vi "Проверка работоспособности.vi"() -> ()   [LabVIEW 2013]
uses:
  IS-95/transmitter/4800/coding(4800).vi
  IS-95/transmitter/common/interleaver.vi
  IS-95/transmitter/9600/coding(9600).vi
  <vilib>/Analysis/baseanly.llb/A x B.vi
  <vilib>/Analysis/baseanly.llb/Real A x B.vi
  IS-95/transmitter/4800/syndrom(4800).vi
  IS-95/transmitter/9600/syndrom(9600).vi
  <vilib>/Analysis/Matrix/Numeric/Conversions/Array To Matrix.vi
  <vilib>/Analysis/Matrix/Numeric/Conversions/Array To Matrix - RA.vi
  <vilib>/ptbypt/Other Functions.llb/Complex Queue PtByPt.vi
panel:
  in  "Номер\nканала":i32
  in  "stop":bool
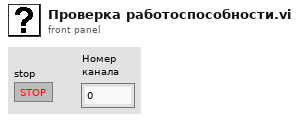
[diagram p1: front panel]
types:
  T1 = cluster{"Amplitude":dbl, "Number":i32, "Frame":bool[], "Type":i32}
  T2 = cluster{"Amplitude":dbl, "Number":i32, "Frame":bool[], "Type":i32}[]
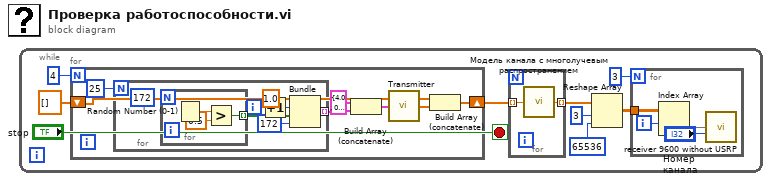
[diagram p0: block diagram]
diagram:
  n1 = while {
    stop <- "stop" stop-if-true
    n2 = for {
      N: 4 -> [_]
      shift-right: [w17] -> w6
      shift-left: cdb[] [] -> [w16]
      n3 = for {
        N: 25 -> [_]
        tunnel: [w25] -> w21 mode=indexing
        i -> [w26]
        n4 = for {
          N: 172 -> [_]
          tunnel: [w30] -> w24 mode=indexing
          n5 = Random Number (0-1)() -> (number: 0 to 1=w32:dbl)
          n6 = Greater?(x=w32, y=0.5) -> (0:w30:bool)
        }
        n7 = Increment(x=w26) -> (x+1=w27:i32)
        n8 = Bundle(1.0, w27, w24, 172) -> (w25:cluster{dbl, i32, bool[], i32})  [unwired: 1 in]
      }
      n9 = Build Array (concatenate)(T1 {"Amplitude"=4.0, "Number"=0, "Frame"=[FALSE, FALSE, FALSE, FALSE, FALSE, FALSE, FALSE, FALSE, FALSE, FALSE, FALSE, FALSE, FALSE, FALSE, FALSE, FALSE, FALSE, FALSE, FALSE, FALSE, FALSE, FALSE, FALSE, FALSE, FALSE, FALSE, FALSE, FALSE, FALSE, FALSE, FALSE, FALSE, FALSE, FALSE, FALSE, FALSE, FALSE, FALSE, FALSE, FALSE, FALSE, FALSE, FALSE, FALSE, FALSE, FALSE, FALSE, FALSE, FALSE, FALSE, FALSE, FALSE, FALSE, FALSE, FALSE, FALSE, FALSE, FALSE, FALSE, FALSE, FALSE, FALSE, FALSE, FALSE, FALSE, FALSE, FALSE, FALSE, FALSE, FALSE, FALSE, FALSE, FALSE, FALSE, FALSE, FALSE, FALSE, FALSE, FALSE, FALSE, FALSE, FALSE, FALSE, FALSE, FALSE, FALSE, FALSE, FALSE, FALSE, FALSE, FALSE, FALSE, FALSE, FALSE, FALSE, FALSE, FALSE, FALSE, FALSE, FALSE, FALSE, FALSE, FALSE, FALSE, FALSE, FALSE, FALSE, FALSE, FALSE, FALSE, FALSE, FALSE, FALSE, FALSE, FALSE, FALSE, FALSE, FALSE, FALSE, FALSE, FALSE, FALSE, FALSE, FALSE, FALSE, FALSE, FALSE, FALSE, FALSE, FALSE, FALSE, FALSE, FALSE, FALSE, FALSE, FALSE, FALSE, FALSE, FALSE, FALSE, FALSE, FALSE, FALSE, FALSE, FALSE, FALSE, FALSE, FALSE, FALSE, FALSE, FALSE, FALSE, FALSE, FALSE, FALSE, FALSE, FALSE, FALSE, FALSE, FALSE, FALSE, FALSE, FALSE, FALSE, FALSE, FALSE, FALSE, FALSE, FALSE, FALSE, FALSE, FALSE], "Type"=172} ("Cluster"), w21) -> (w19:T2)
      n10 = call "Transmitter.vi"("CHANNELS"=w19) -> ("x + iy"=w18:cdb[])  [unwired: 14 in]
      n11 = Build Array (concatenate)(w16, w18) -> (w17:cdb[])
    }
    n12 = for {
      tunnel: w6 -> [w15] mode=indexing
      tunnel: [w14] -> w7 mode=indexing
      n13 = call "Модель канала с многолучевым распространением.vi"("Выборка\nс передатчика"=w15) -> ("Выборка \nс канала"=w14:cdb)  [unwired: 14 in]
    }
    n14 = Reshape Array(w7, 3 ("dimension size"), 65536 ("dimension size")) -> (w8:cdb[][])
    n15 = for {
      N: 3 -> [_]
      tunnel: w8 -> [w13]
      i -> [w10]
      n16 = Index Array(array=w13, index (row)=w10) -> (element=w12:cdb[])  [unwired: 1 in]
      n17 = call "receiver 9600 without USRP.vi"("coming\ndata"=w12, "Номер\nканала"="Номер\nканала") -> ()  [unwired: 14 in]
    }
  }
